vi "Update Dependencies.vi"(7 "Logger":refnum<class "Logger.lvclass">, 8 "error in (no error)":errorcluster, 11 "PackageAbstract in":refnum<class "PackageAbstract.lvclass">) -> (0 "error out":errorcluster, 3 "PackageAbstract out":refnum<class "PackageAbstract.lvclass">)   [LabVIEW 2020, in "GPack.lvlib" / "PackageAbstract.lvclass"]
uses:
  PackageAbstract.lvclass
  C:/dev/lv20CE/lv-gpack/GPack/Package/Package.lvclass
  Logger/Logger.lvclass
  PackageAbstract.lvclass/PackageAbstract.ctl
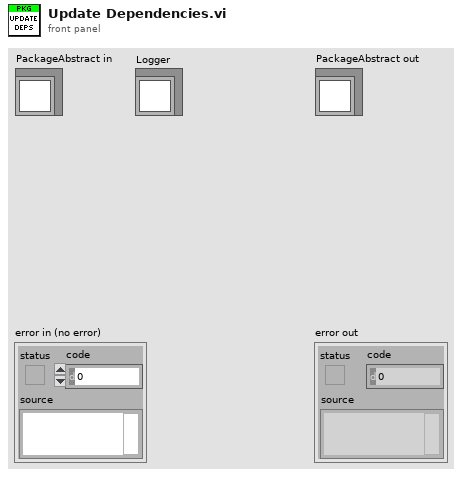
[diagram p1: front panel]
types:
  T1 = typedef "GPack.lvlib/Dependency.ctl" = cluster{"Info":T2, "Path":path}
  T2 = typedef "GPack.lvlib/Package Info.ctl" = cluster{"Name":string, "Type":string, "Host":string, "Path":string, "Branch":string, "Version":string, "License":string}
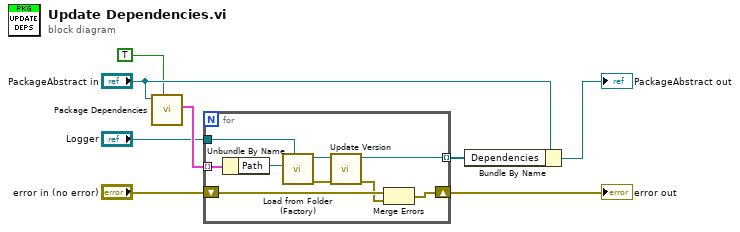
[diagram p0: block diagram]
diagram:
  n1 = call-dynamic "Package Dependencies.vi"("Absolute Path (F)"=TRUE, "PackageAbstract in"="PackageAbstract in") -> ("Dependencies"=w6:T1[])  [unwired: 8 in, 1 out]
  n2 = for {
    tunnel: "Logger" -> [w15]
    tunnel: w6 -> [w17] mode=indexing
    shift-right: [w9] -> w3
    shift-left: "error in (no error)" -> [w11]
    tunnel: [w12] -> w1 mode=indexing
    n3 = Unbundle By Name(w17) -> ("Path"=w16:path)
    n4 = call "Load from Folder (Factory).vi"("Logger"=w15, "Folder"=w16) -> ("error out"=w13:errorcluster, "PackageAbstract out"=w14:refnum<class "PackageAbstract.lvclass">)  [unwired: 8 in]
    n5 = call-dynamic "Update Version.vi"("error in (no error)"=w13, "Package in"=w14) -> ("error out"=w10:errorcluster, "Package out"=w12:refnum<class "PackageAbstract.lvclass">)  [unwired: 8 in]
    n6 = Merge Errors(w11, w10) -> (w9:errorcluster)
  }
  "error out" <- w3
  n7 = Bundle By Name(cluster="PackageAbstract in", "Dependencies"=w1) -> (→"PackageAbstract out":refnum<class "PackageAbstract.lvclass">)
